vi "Report error from STATUS.vi"(8 "error in":errorcluster, 11 "payload":u8[](array[numeric])) -> (0 "error out":errorcluster)   [LabVIEW 2020, in "NI_SFTP.lvlib"]
uses:
  <vilib>/net/SFTP/NI_SFTP.lvlib
  <vilib>/net/SSH/NI_SSH.lvlib
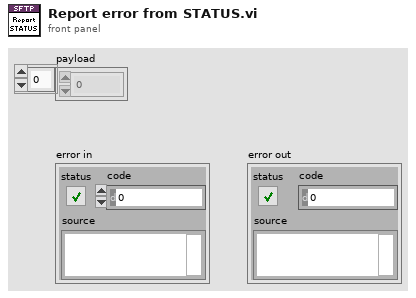
[diagram p1: front panel]
types:
  T1 = typedef "NI_SFTP.lvlib/Low Level Connection.lvclass/Status Code.ctl" = enum32{"SSH_FX_OK", "SSH_FX_EOF", "SSH_FX_NO_SUCH_FILE", "SSH_FX_PERMISSION_DENIED", "SSH_FX_FAILURE", "SSH_FX_BAD_MESSAGE", "SSH_FX_OP_UNSUPPORTED"}
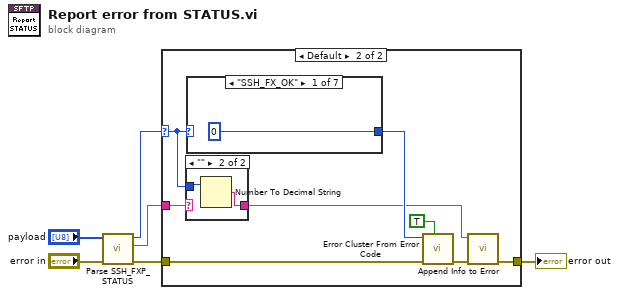
[diagram p0: block diagram]
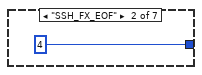
[diagram p4: hidden frame]
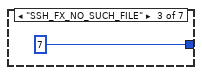
[diagram p5: hidden frame]
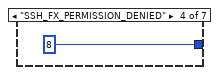
[diagram p6: hidden frame]
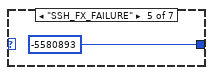
[diagram p7: hidden frame]
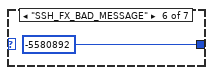
[diagram p8: hidden frame]
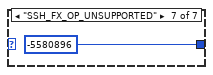
[diagram p9: hidden frame]
diagram:
  n1 = call <vilib>:"Parse SSH_FXP_STATUS.vi"("error in"="error in", "payload"="payload") -> ("error out"=w4:errorcluster, "error message"=w6:string, "error/status code"=w1:T1)  [unwired: 6 in, 1 out]
  n2 = case shown="Default" w1 {
    selector: w1 -> [_ w11]
    tunnel: w6 -> [_ w12]
    tunnel: [w7 w9] -> w5
    tunnel: w4 -> [w7 w14]
    frame "SSH_FX_OK" {
    }
    frame Default {
      n3 = case shown="\"\"" w12 {
        selector: w12 -> [w16 _]
        tunnel: [w16 w18] -> w8
        tunnel: w11 -> [_ w17]
        frame Default {
        }
        frame "" {
          n4 = Number To Decimal String(number=w17) -> (decimal integer string=w18:string)  [unwired: 1 in]
        }
      }
      n5 = case shown="\"SSH_FX_OK\"" w11 {
        tunnel: [0 ("error code (0)") 4 ("EOF") 7 ("error code (0)") 8 ("error code (0)") -5580893 ("error code (0)") -5580892 ("error code (0)") -5580896 ("error code (0)")] -> w13
        frame "SSH_FX_OK" {
        }
        frame "SSH_FX_EOF" {
        }
        frame "SSH_FX_NO_SUCH_FILE" {
        }
        frame "SSH_FX_PERMISSION_DENIED" {
        }
        frame "SSH_FX_FAILURE" {
        }
        frame "SSH_FX_BAD_MESSAGE" {
        }
        frame "SSH_FX_OP_UNSUPPORTED" {
        }
      }
      n6 = call <vilib>:"Error Cluster From Error Code.vi"("show call chain? (False)"=TRUE, "error in (no error)"=w14, "error code (0)"=w13) -> ("error out"=w10:errorcluster)  [unwired: 6 in]
      n7 = call <vilib>:"Append Info to Error.vi"("error in (no error)"=w10, "additional info"=w8) -> ("error out"=w9:errorcluster)  [unwired: 9 in]
    }
  }
  "error out" <- w5
